vi "Disabled.vi"(7 "Robot Mode":T2, 10 "Match Info":T1={"Autonomous Elapsed Seconds"=0.0, "TeleOp Elapsed Seconds"=0.0, "Disabled Elapsed Seconds"=0.0, "Visited Autonomous"=FALSE, "Visited TeleOp"=FALSE, "Visited Disabled"=FALSE, "Autonomous Settings"={"Autonomous Style"=enum."Independent", "VI Refnum"=refnum}}, 11 "Call Context":T3) -> ()   [LabVIEW 2019]
doc: "This VI is called each time a disabled packet is received from the DS. It is often used to prepare for the next robot mode, to calibrate sensors, etc."
uses:
  <vilib>/Rock Robotics/WPI/DriverStation/WPI_DriverStationDerivedRobotMode.ctl
  <vilib>/Rock Robotics/WPI/DriverStation/WPI_DriverStationRobotMode2.ctl
  <vilib>/Rock Robotics/WPI/DriverStation/WPI_DriverStationMatch Info.ctl
  RobotGlobal.vi
  Classes/DriveOld/Drive.lvclass
  Classes/Elevator/Elevator.lvclass
  Classes/Vision/Vision.lvclass
panel:
  out "error out":errorcluster
  in  "error in (no error)":errorcluster
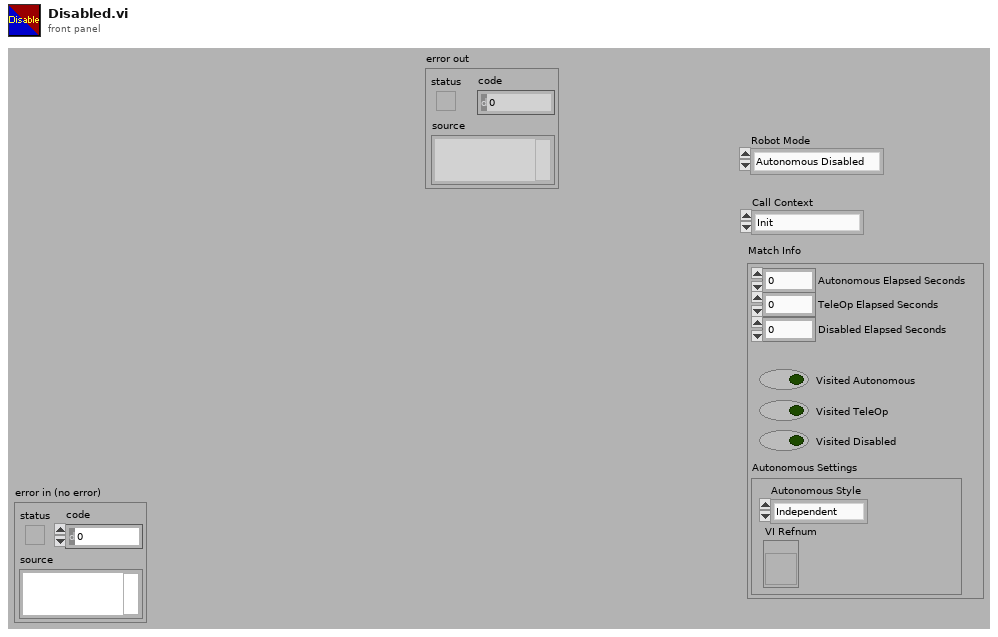
[diagram p1: front panel]
types:
  T1 = typedef "WPI_DriverStationMatch Info.ctl" = cluster{"Autonomous Elapsed Seconds":dbl, "TeleOp Elapsed Seconds":dbl, "Disabled Elapsed Seconds":dbl, "Visited Autonomous":bool, "Visited TeleOp":bool, "Visited Disabled":bool, "Autonomous Settings":cluster{"Autonomous Style":enum16{"Iterative", "Independent"}, "VI Refnum":refnum<vi>}}
  T2 = typedef "WPI_DriverStationRobotMode2.ctl" = enum16{"Autonomous Disabled", "Autonomous Enabled", "Teleop Disabled", "Teleop Enabled", "Disconnected", "Finish", "Test Disabled", "Test Enabled", "Emergency Stopped"}
  T3 = typedef "WPI_DriverStationDerivedRobotMode.ctl" = enum16{"Init", "Execute", "Stop"}
  T4 = typedef "RobotObjects.ctl" = cluster{"Drive.lvclass":refnum<class "Tank Drive.lvclass">, "Pneumatics.lvclass":refnum<class "Pneumatics.lvclass">, "Vision.lvclass":refnum<class "Vision.lvclass">, "Joysticks.lvclass":refnum<class "Joysticks.lvclass">, "Elevator.lvclass":refnum<class "Elevator.lvclass">, "Hatch.lvclass":refnum<class "Hatch.lvclass">, "Cargo.lvclass":refnum<class "Cargo.lvclass">, "DriveOld.lvclass":refnum<class "Drive.lvclass">, "Robot.lvclass":refnum<class "Robot.lvclass">, "Control Panel.lvclass":refnum<class "Control Panel.lvclass">, "Climber.lvclass":refnum<class "Climber.lvclass">, "Turret.lvlib:Turret.lvclass":refnum<class "Turret.lvclass">, "Power Cell Handler.lvclass":refnum<class "Power Cell Handler.lvclass">}
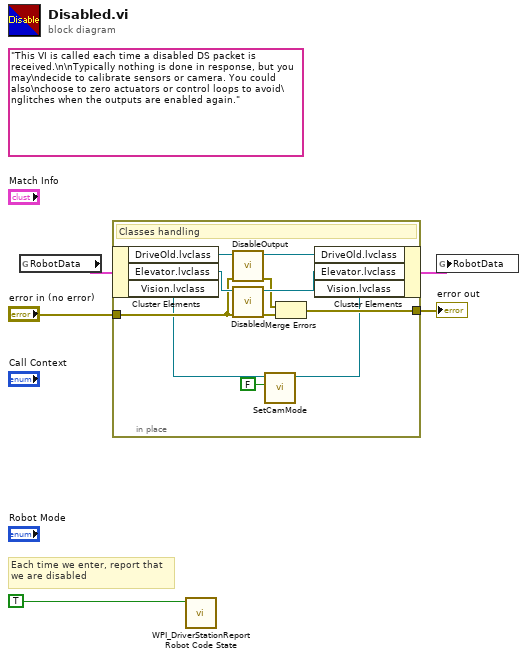
[diagram p0: block diagram]
diagram:
  (unwired) "This VI is called each time a disabled DS packet is received.\n\nTypically nothing is done in response, but you may\ndecide to calibrate sensors or camera. You could also\nchoose to zero actuators or control loops to avoid\nglitches when the outputs are enabled again."
  # "Each time we enter, report that\nwe are disabled"
  n1 = global read "RobotGlobal.vi" "RobotData"() -> (w4:T4)
  n2 = in-place {
    in-place-border: "error in (no error)" -> [w9]
    in-place-border: [w12] -> w1
    # "Classes handling"
    n3 = in-place-cluster #1(w4) -> ("DriveOld.lvclass"=w16:refnum<class "Drive.lvclass">, "Elevator.lvclass"=w14:refnum<class "Elevator.lvclass">, "Vision.lvclass"=w8:refnum<class "Vision.lvclass">)
    n4 = call-dynamic "DisableOutput.vi"("error in (no error)"=w9, "Drive in"=w16) -> ("error out"=w10:errorcluster, "Drive out"=w15:refnum<class "Drive.lvclass">)  [unwired: 8 in]
    n5 = call-dynamic "Disabled.vi"("error in (no error)"=w9, "Elevator in"=w14) -> ("error out"=w11:errorcluster, "Elevator out"=w13:refnum<class "Elevator.lvclass">)  [unwired: 8 in]
    n6 = call "SetCamMode.vi"("Vision.lvlib:Vision.lvclass"=w8, "Vision Processing?"=FALSE) -> ("Vision.lvlib:Vision.lvclass"=w7:refnum<class "Vision.lvclass">)  [unwired: 7 in, 1 out]
    n7 = Merge Errors(w10, w11) -> (w12:errorcluster)
    n8 = in-place-cluster #1("DriveOld.lvclass"=w15, "Elevator.lvclass"=w13, "Vision.lvclass"=w7) -> (w3:T4)
  }
  "error out" <- w1
  n9 = call <vilib>:"WPI_DriverStationReport Robot Code State.vi"("Disabled"=TRUE ("Autonomous")) -> ()  [unwired: 10 in, 1 out]
  n10 = global write "RobotGlobal.vi" "RobotData"(w3) -> ()
